vi "Populate VS channel control - Any Channel by Path Array.vi"(7 "DisplayFilter":u8(ring)=7 items=["K_CHAN_R", "K_CHAN_W", "K_CHAN_RW", "K_CHAN_VOLT", "K_CHAN_FAULT", "K_ALL", "K_CUSTOM", "K_CHAN_R_VIS", "K_CHAN_W_VIS", "K_CHAN_RW_VIS", "K_CHAN_VOLT_VIS", "K_CHAN_FAULT_VIS"], 8 "error in (no error)":errorcluster, 9 "Path Array In":string[](array[string]), 10 "NIVS.System Definition Root":refnum<k24>, 11 ".NET Refnum in":refnum<k24>) -> (0 "error out":errorcluster, 3 ".NET Refnum out":refnum<k24>)   [LabVIEW 2013]
uses:
  NationalInstruments.VeriStand.SystemStorageUI
  NationalInstruments.VeriStand.SystemStorage
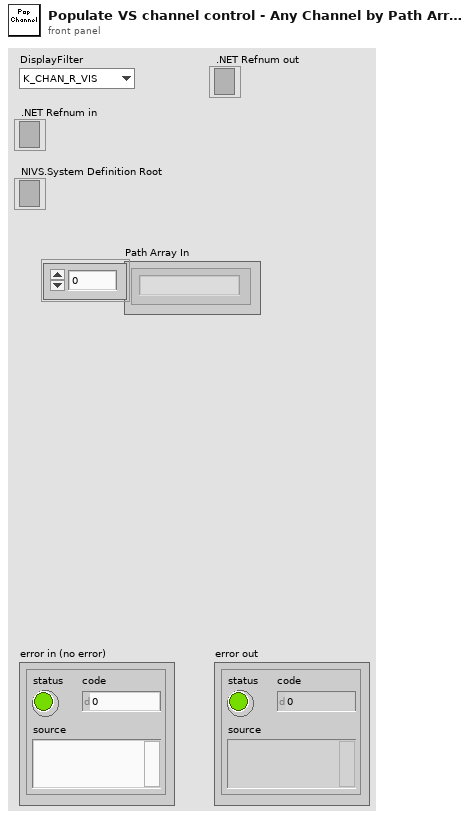
[diagram p1: front panel]
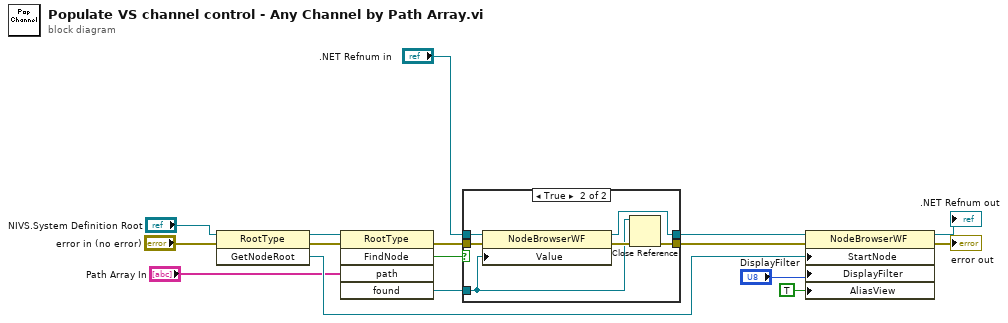
[diagram p0: block diagram]
diagram:
  n1 = invoke class="RootType" method="GetNodeRoot"(reference="NIVS.System Definition Root", error in="error in (no error)") -> (reference out=w6:refnum<k24>, error out=w5:errorcluster, "GetNodeRoot"=w2:refnum<k24>)  [unwired: 1 in]
  n2 = invoke class="RootType" method="FindNode"(reference=w6, error in=w5, "path"="Path Array In") -> (error out=w12:errorcluster, "FindNode"=w14:bool, "found"=w11:refnum<k24>)  [unwired: 2 in, 2 out]
  n3 = case shown="True" w14 {
    tunnel: w11 -> [_ w19]
    tunnel: w12 -> [w18 w20]
    tunnel: [w18 w23] -> w13
    tunnel: ".NET Refnum in" -> [w17 w22]
    tunnel: [w17 w21] -> w15
    frame False {
    }
    frame True {
      n4 = property class="NodeBrowserWF"(reference=w22, error in=w20, "Value"=w19) -> (reference out=w21:refnum<k24>, error out=w24:errorcluster)
      n5 = Close Reference(reference=w19, error in (no error)=w24) -> (error out=w23:errorcluster)
    }
  }
  n6 = property class="NodeBrowserWF"(reference=w15, error in=w13, "StartNode"=w2, "DisplayFilter"="DisplayFilter", "AliasView"=TRUE) -> (reference out=→".NET Refnum out":refnum<k24>, error out=→"error out":errorcluster)
